vi "Edit_Raw_DF_Header_Manual.vi"() -> ()   [LabVIEW 2010]
uses:
  Anemometry/Anemometry Sub Vis/Controls/File_Selector_Type.ctl
panel:
  out "Currently File Number":i32
  out "No of Unfound files":i32
  out "Unfound Files":path[](array[path])
  out "File Number":i32
  out "Current case":string
  out "Currently Editting":path
  in  "Variables and values":string[][](array[string])=[["BSA 1 Extra_Info", "Tunnel"], ["BSA 2 Extra_Info", "Tunnel"]]
  out "No of Files to edit":i32
  in  "Previous Choice":path
  in  "Search String":string
  in  "At Dialog Prompt for Editting Raw data files":T1
  # "Variables to Insert/Edit"
  # "Desired Values"
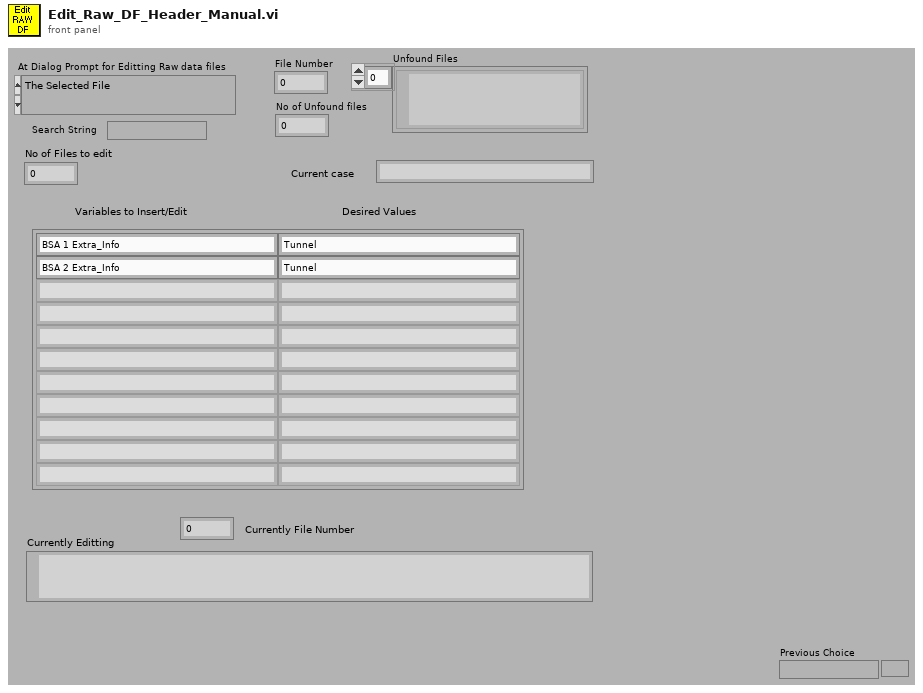
[diagram p1: front panel]
types:
  T1 = typedef "File_Selector_Type.ctl" = enum16{"The Selected File", "The Selected Folder", "Files containing the search string in the selected folder", "All files listed in selected file"}
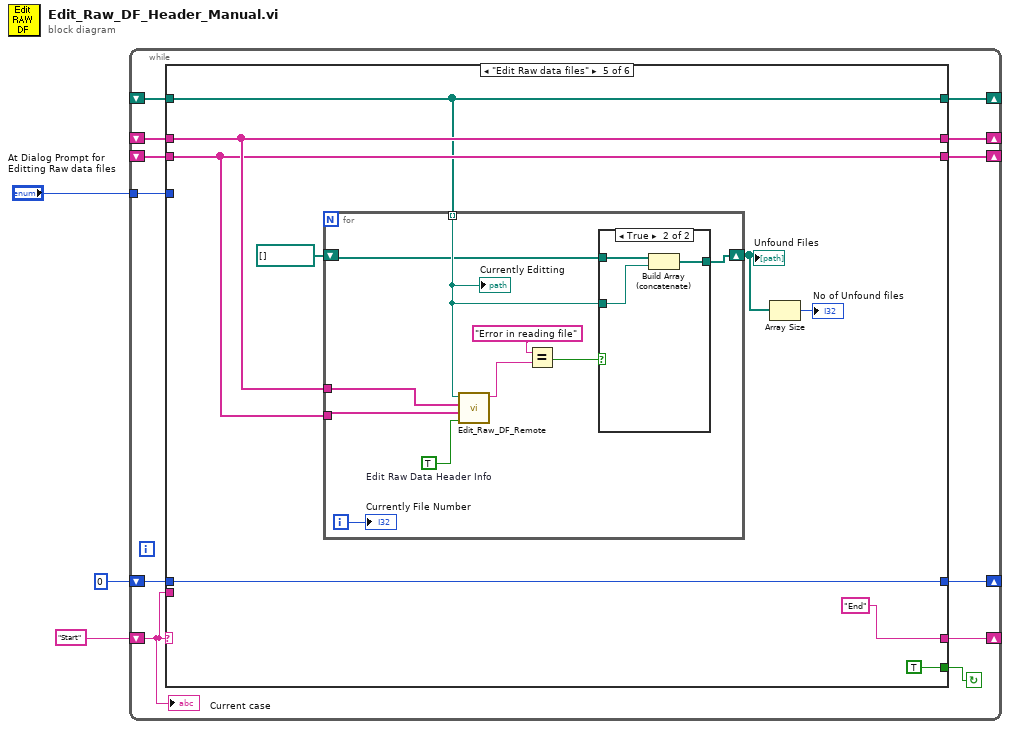
[diagram p0: block diagram]
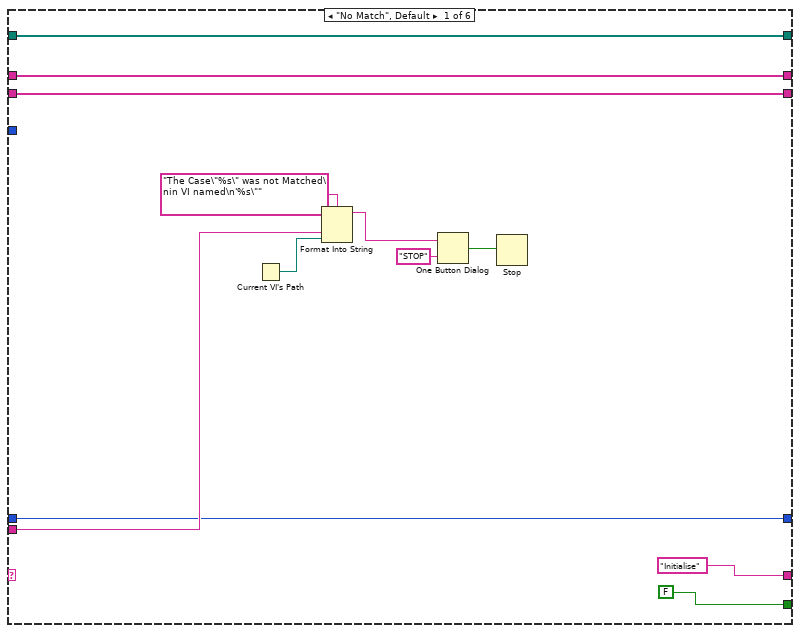
[diagram p2: hidden frame]
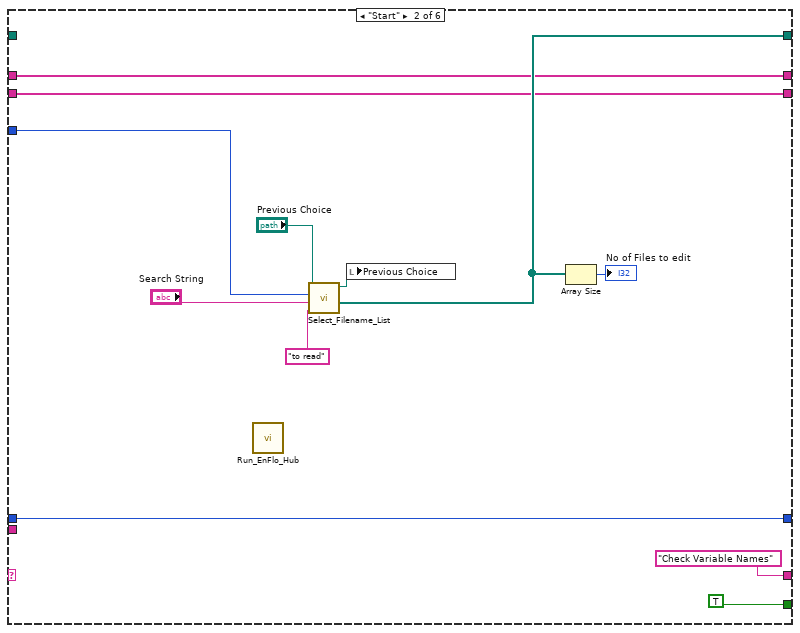
[diagram p3: hidden frame]
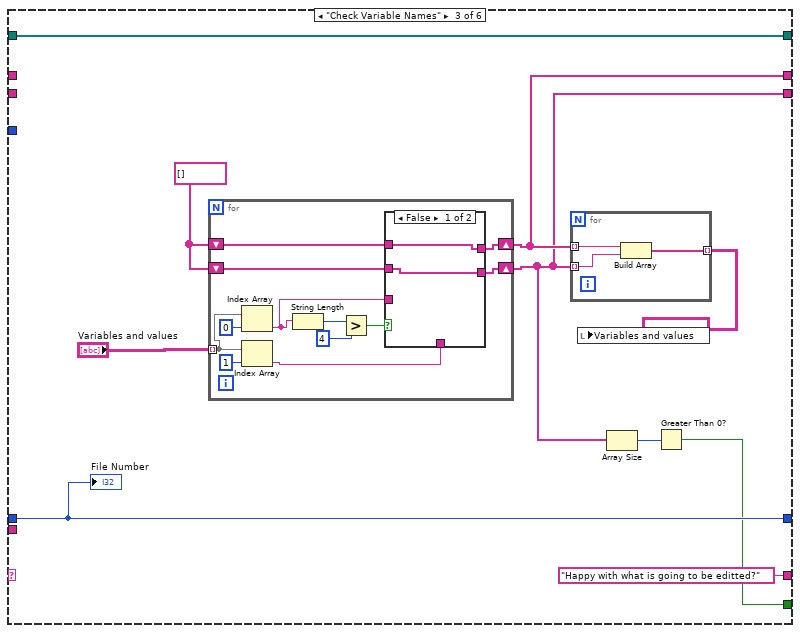
[diagram p4: hidden frame]
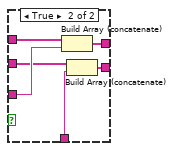
[diagram p5: hidden frame]
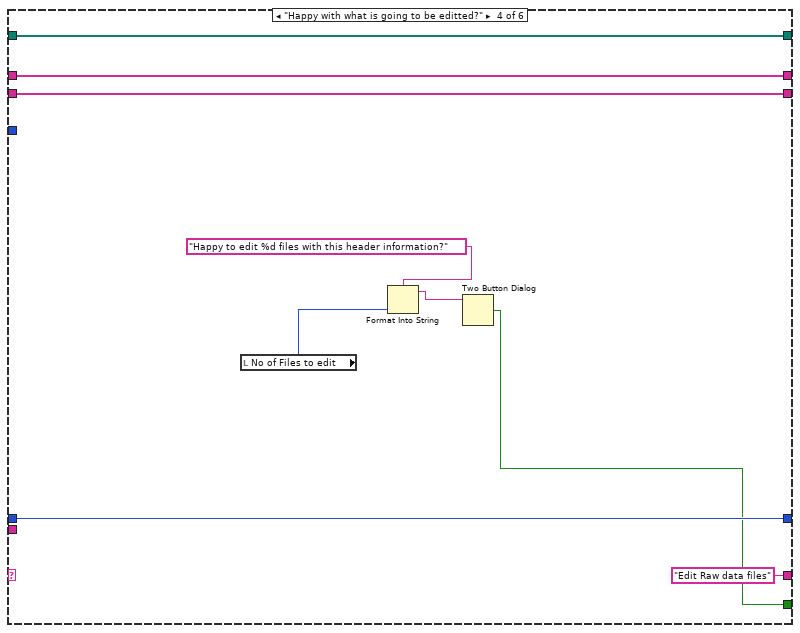
[diagram p6: hidden frame]
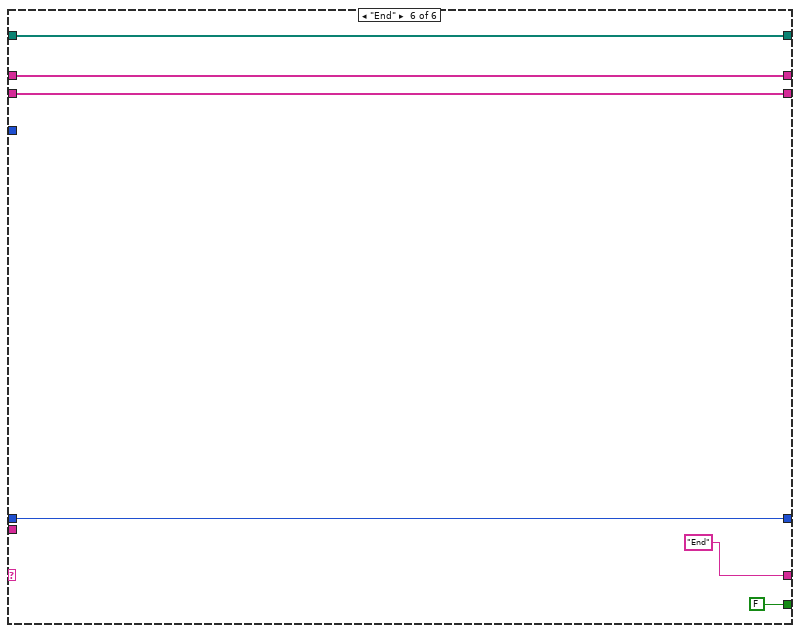
[diagram p8: hidden frame]
diagram:
  n1 = while {
    shift-left: "Start" -> [w13]
    shift-right: [w14] -> _
    shift-right: [w11] -> _
    shift-left: _ -> [w12]
    tunnel: "At Dialog Prompt for Editting Raw data files" -> [w10]
    shift-right: [w4] -> _
    shift-left: 0 -> [w9]
    shift-right: [w8] -> _
    shift-left: _ -> [w7]
    shift-right: [w5] -> _
    shift-left: _ -> [w6]
    stop <- w15 continue-if-true
    n2 = case shown="\"Edit Raw data files\"" w13 {
      tunnel: [FALSE TRUE w41 w79 TRUE ("T button?") FALSE ("T button?")] -> w15
      tunnel: ["Initialise" "Check Variable Names" "Happy with what is going to be editted?" "Edit Raw data files" "End" "End"] -> w14
      tunnel: w13 -> [w22 _ _ _ _ _]
      tunnel: w12 -> [w19 _ w49 w81 w82 w110]
      tunnel: [w19 w32 w49 w81 w82 w110] -> w11
      tunnel: w10 -> [_ w38 _ _ _ _]
      tunnel: w9 -> [w16 w30 w48 w80 w89 w106]
      tunnel: [w18 w29 w44 w77 w87 w108] -> w8
      tunnel: w7 -> [w18 w29 _ w77 w87 w108]
      tunnel: w6 -> [w17 w28 _ w76 w86 w109]
      tunnel: [w17 w28 w43 w76 w86 w109] -> w5
      tunnel: [w16 w30 w48 w80 w89 w106] -> w4
      frame "No Match", Default {
        n3 = Current VI's Path() -> (path=w21:path)
        n4 = Format Into String(format string="The Case\"%s\" was not Matched\nin VI named\n'%s\"" ("Format String"), w22, w21) -> (resulting string=w25:string)  [unwired: 2 in, 1 out]
        n5 = One Button Dialog(message=w25, button name ("OK")="STOP") -> (true=w23:bool)
        n6 = Stop(stop? (T)=w23) -> ()
      }
      frame "Start" {
        n7 = call "Run_EnFlo_Hub.vi"() -> ()  [unwired: 8 in]
        n8 = call "Select_Filename_List.vi"("File Type"="to read", "Search String"="Search String", "At Dialog Prompt Post Process"=w38, "Previous Choice"="Previous Choice") -> ("Selected files"=w32:path[], "Choosen path"=w34:path)  [unwired: 2 in, 1 out]
        n9 = local write "Previous Choice"(w34) -> ()
        n10 = Array Size(array=w32) -> (size(s)=→"No of Files to edit":i32)
      }
      frame "Check Variable Names" {
        w46 = string[] []
        n11 = for {
          shift-right: [w57] -> w44
          shift-left: w46 -> [w58]
          shift-right: [w53] -> w43
          shift-left: w46 -> [w55]
          tunnel: "Variables and values" -> [w62] mode=indexing
          n12 = Index Array(array=w62, index=0) -> (element=w56:string)
          n13 = Index Array(array=w62, index=1) -> (element=w54:string)
          n14 = String Length(string=w56) -> (length=w61:i32)
          n15 = Greater?(x=w61, y=4) -> (0:w59:bool)
          n16 = case shown="False" w59 {
            tunnel: w58 -> [w66 w72]
            tunnel: [w66 w70] -> w57
            tunnel: w56 -> [_ w71]
            tunnel: w55 -> [w65 w69]
            tunnel: w54 -> [_ w68]
            tunnel: [w65 w67] -> w53
            frame False {
            }
            frame True {
              n17 = Build Array (concatenate)(w72, w71) -> (w70:string[])
              n18 = Build Array (concatenate)(w69, w68) -> (w67:string[])
            }
          }
        }
        n19 = for {
          tunnel: w44 -> [w52] mode=indexing
          tunnel: w43 -> [w51] mode=indexing
          tunnel: [w50] -> w45 mode=indexing
          n20 = Build Array(w52, w51) -> (w50:string[])
        }
        n21 = local write "Variables and values"(w45) -> ()
        n22 = Array Size(array=w43) -> (size(s)=w42:i32)
        n23 = Greater Than 0?(x=w42) -> (x > 0?=w41:bool)
        "File Number" <- w48
      }
      frame "Happy with what is going to be editted?" {
        n24 = local read "No of Files to edit"() -> (w75:i32)
        n25 = Format Into String(format string="Happy to edit %d files with this header information?" ("message"), w75) -> (resulting string=w73:string)  [unwired: 2 in, 1 out]
        n26 = Two Button Dialog(message=w73) -> (T button?=w79:bool)  [unwired: 2 in]
      }
      frame "Edit Raw data files" {
        n27 = for {
          tunnel: w87 -> [w100]
          tunnel: w86 -> [w98]
          tunnel: w82 -> [w94] mode=indexing
          shift-right: [w92] -> w85
          shift-left: path[] [] -> [w93]
          i -> [w91]
          w99 = TRUE  # Edit Raw Data Header Info
          n28 = call "Edit_Raw_DF_Remote.vi"("Edit Raw Data Header Info"=w99, "New Values In"=w98, "New Chs In"=w100, "Current Filename"=w94) -> ("Filetype"=w96:string)  [unwired: 3 out]
          n29 = Equal?(x="Error in reading file", y=w96) -> (x = y?=w95:bool)
          n30 = case shown="True" w95 {
            tunnel: w94 -> [_ w104]
            tunnel: w93 -> [w101 w103]
            tunnel: [w101 w102] -> w92
            frame False {
            }
            frame True {
              n31 = Build Array (concatenate)(w103, w104) -> (w102:path[])
            }
          }
          "Currently Editting" <- w94
          "Currently File Number" <- w91
        }
        "Unfound Files" <- w85
        n32 = Array Size(array=w85) -> (size(s)=→"No of Unfound files":i32)
      }
      frame "End" {
      }
    }
    "Current case" <- w13
  }
